vi "系统交互.vi"   [LabVIEW 2016]
uses:
  <vilib>/Utility/config.llb/NI_LVConfig.lvlib
types:
  T1 = typedef "系统交互.ctl" = cluster{"运行模式":enum16{"维护模式", "常规模式", "应急模式", "质控模式"}, "运行间隔":i16, "流程运行中":bool, "自动运行启动参数":T2, "SYSTEM Interface.总磷总氮类型":enum16{"单模块", "总磷总氮二合一模块", "氨氮总磷二合一模块"}, "多参数运行间隔":i16, "配水时间":dbl, "沉淀时间":dbl, "清洗时间":dbl, "关键参数改变":bool}
  T2 = typedef "启动参数.ctl" = cluster{"氨氮":bool, "总磷":bool, "总氮":bool, "多参数":bool, "CODmn":bool, "CODCr":bool, "氟化物":bool, "超标留样启用":bool}
  T3 = cluster{"运行模式":enum16{"维护模式", "常规模式", "应急模式", "质控模式"}, "质控频次":enum16{"关闭", "每天", "星期一", "星期二", "星期三", "星期四", "星期五", "星期六", "星期日"}, "空白核查时间":u16, "跨度核查时间":u16, "多参数测试间隔":u16, "湿化学测试间隔":u16}
  T4 = typedef "NI_LVConfig.lvlib/Config Data RefNum.ctl" = refnum<k1>
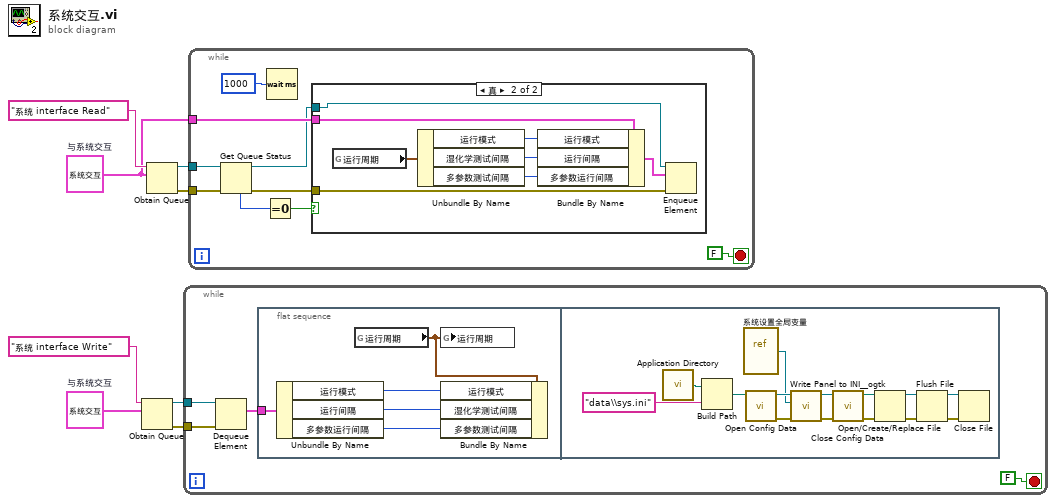
[diagram p0: block diagram]
diagram:
  w4 = T1 {"运行模式"=enum."维护模式", "运行间隔"=4, "流程运行中"=FALSE, "自动运行启动参数"={"氨氮"=FALSE, "总磷"=FALSE, "总氮"=FALSE, "多参数"=FALSE, "CODmn"=FALSE, "CODCr"=FALSE, "氟化物"=FALSE, "超标留样启用"=FALSE}, "SYSTEM Interface.总磷总氮类型"=enum."单模块", "多参数运行间隔"=4, "配水时间"=0.0, "沉淀时间"=0.0, "清洗时间"=0.0, "关键参数改变"=FALSE}  # 与系统交互
  w5 = T1 {"运行模式"=enum."维护模式", "运行间隔"=4, "流程运行中"=FALSE, "自动运行启动参数"={"氨氮"=FALSE, "总磷"=FALSE, "总氮"=FALSE, "多参数"=FALSE, "CODmn"=FALSE, "CODCr"=FALSE, "氟化物"=FALSE, "超标留样启用"=FALSE}, "SYSTEM Interface.总磷总氮类型"=enum."单模块", "多参数运行间隔"=4, "配水时间"=0.0, "沉淀时间"=0.0, "清洗时间"=0.0, "关键参数改变"=FALSE}  # 与系统交互
  n1 = Obtain Queue(name (unnamed)="系统 interface Write" ("写入方名称"), element data type=w4) -> (queue out=w2:refnum<queue>, error out=w3:errorcluster)  [unwired: 3 in, 1 out]
  n2 = Obtain Queue(name (unnamed)="系统 interface Read" ("写入方名称"), element data type=w5) -> (queue out=w7:refnum<queue>, error out=w6:errorcluster)  [unwired: 3 in, 1 out]
  n3 = while {
    tunnel: w2 -> [w11]
    tunnel: w3 -> [w10]
    stop <- FALSE stop-if-true
    n4 = Dequeue Element(queue=w11, error in (no error)=w10) -> (element=w9:T1)  [unwired: 1 in, 3 out]
    n5 = flat-sequence {
      tunnel: w9 -> [w17]
      frame #0 {
        n6 = Unbundle By Name(w17) -> ("运行模式"=w16:enum16{"维护模式", "常规模式", "应急模式", "质控模式"}, "运行间隔"=w15:i16, "多参数运行间隔"=w14:i16)
        n7 = global read "系统设置全局变量.vi" "运行周期"() -> (w13:T3)
        n8 = global write "系统设置全局变量.vi" "运行周期"(w13) -> ()
        n9 = Bundle By Name(cluster=w13, "运行模式"=w16, "湿化学测试间隔"=w15, "多参数测试间隔"=w14) -> ()  [unwired: 1 out]
      }
      frame #1 {
        n10 = call <vilib>:"Application Directory.vi"() -> ("Application Directory"=w31:path)
        n11 = Build Path(base path=w31, name or relative path="data\\sys.ini" ("名称或相对路径")) -> (appended path=w29:path)
        n12 = vi-ref "系统设置全局变量.vi"() -> (w27:refnum<vi>)
        n13 = call <vilib>:"Open Config Data.vi"("configuration file path"=w29) -> ("error out"=w25:errorcluster, "refnum"=w28:T4)  [unwired: 8 in, 1 out]
        n14 = call <userlib>:"Write Panel to INI__ogtk.vi"("error in (no error)"=w25, "VI ref"=w27, "refnum"=w28) -> ("error out"=w24:errorcluster, "refnum out"=w26:T4)  [unwired: 7 in]
        n15 = call <vilib>:"Close Config Data.vi"("error in (no error)"=w24, "refnum"=w26) -> ("error out"=w19:errorcluster, "file path"=w18:path)  [unwired: 8 in]
        n16 = Open/Create/Replace File(file path (use dialog)=w18, error in=w19) -> (refnum out=w22:refnum<file>, error out=w23:errorcluster)  [unwired: 4 in, 1 out]
        n17 = Flush File(refnum=w22, error in=w23) -> (refnum out=w21:refnum<file>, error out=w20:errorcluster)
        n18 = Close File(refnum=w21, error in=w20) -> ()  [unwired: 2 out]
      }
    }
  }
  n19 = while {
    tunnel: w7 -> [w38]
    tunnel: w6 -> [w34]
    tunnel: w5 -> [w37]
    stop <- FALSE stop-if-true
    n20 = Get Queue Status(queue=w38, error in (no error)=w34) -> (queue out=w36:refnum<queue>, error out=w32:errorcluster, # elements in queue=w35:i32)  [unwired: 1 in, 5 out]
    n21 = Equal To 0?(x=w35) -> (x = 0?=w33:bool)
    n22 = Wait (ms)(milliseconds to wait=u32 1000 ("等待时间（毫秒）")) -> ()  [unwired: 1 out]
    n23 = case shown="真" w33 {
      tunnel: w37 -> [_ w48]
      tunnel: w36 -> [_ w46]
      tunnel: w32 -> [_ w45]
      frame False {
      }
      frame True {
        n24 = global read "系统设置全局变量.vi" "运行周期"() -> (w44:T3)
        n25 = Unbundle By Name(w44) -> ("运行模式"=w43:enum16{"维护模式", "常规模式", "应急模式", "质控模式"}, "湿化学测试间隔"=w42:u16, "多参数测试间隔"=w41:u16)
        n26 = Bundle By Name(cluster=w48, "运行模式"=w43, "运行间隔"=w42, "多参数运行间隔"=w41) -> (w47:T1)
        n27 = Enqueue Element(queue=w46, element=w47, error in (no error)=w45) -> ()  [unwired: 1 in, 3 out]
      }
    }
  }
